vi "New.vi"(5 "Abort Wait Reference 2":refnum<vi>, 7 "Abort Wait Reference":refnum<vi>, 8 "error in (no error)":errorcluster, 9 "Wait for Config Total Time [ms]":i32=1000, 10 "Wait for Config Timeout [ms]":i32=20, 11 "Connection Settings":T1={"IP-address"="150.106.171.173", "Port"="5011", "ID Code"=1001}) -> (0 "error out":errorcluster, 3 "Phasor Data Concentrator out":refnum<class "Phasor Data Concentrator.lvclass">)   [LabVIEW 2013, in "PMU Recorder Light.lvlib" / "Phasor Data Concentrator.lvclass"]
uses:
  Phasor Data Concentrator.lvclass
  Statnett C37.118 DLL/Statnett C37.118 DLL.lvclass
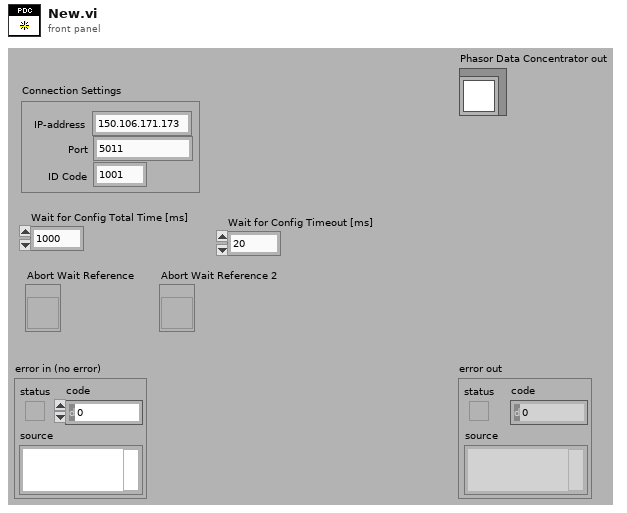
[diagram p1: front panel]
types:
  T1 = cluster{"IP-address":string, "Port":string, "ID Code":u32}
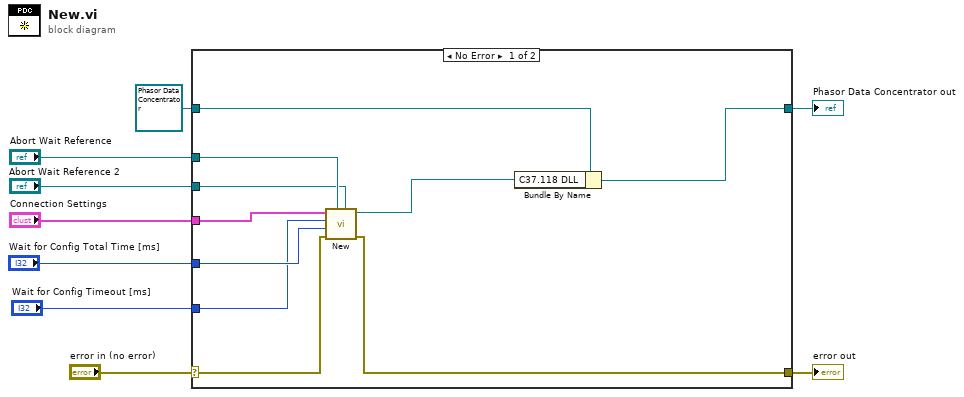
[diagram p0: block diagram]
diagram:
  n1 = case shown="No Error" "error in (no error)" {
    selector: "error in (no error)" -> [w17 w21]
    tunnel: [w16 w21] -> w8
    tunnel: [w13 w20] -> w7
    tunnel: refnum<class "Phasor Data Concentrator.lvclass"> refnum ("Phasor Data Concentrator in") -> [w14 w20]
    tunnel: "Connection Settings" -> [w12 _]
    tunnel: "Wait for Config Total Time [ms]" -> [w18 _]
    tunnel: "Abort Wait Reference" -> [w19 _]
    tunnel: "Wait for Config Timeout [ms]" -> [w11 _]
    tunnel: "Abort Wait Reference 2" -> [w10 _]
    frame No Error {
      n2 = call "New.vi"("Abort Wait Reference 2"=w10, "Abort Wait Reference"=w19, "error in (no error)"=w17, "Wait for Configuration Total Time [ms]"=w18, "Wait for Configuration Timeout [ms]"=w11, "Connection Settings"=w12) -> ("error out"=w16:errorcluster, "Statnett C37.118 DLL out"=w15:refnum<class "Statnett C37.118 DLL.lvclass">)  [unwired: 4 in]
      n3 = Bundle By Name(cluster=w14, "C37.118 DLL"=w15) -> (w13:refnum<class "Phasor Data Concentrator.lvclass">)
    }
    frame Error {
    }
  }
  "error out" <- w8
  "Phasor Data Concentrator out" <- w7
